vi "VLC - Get Program Location (path).vi"(11 "error in (no error)":errorcluster) -> (6 "VLC path":string, 15 "error out":errorcluster)   [LabVIEW 2016]
uses:
  <vilib>/registry/registry.llb/Registry RtKey.ctl
  <vilib>/registry/registry.llb/Registry SAM.ctl
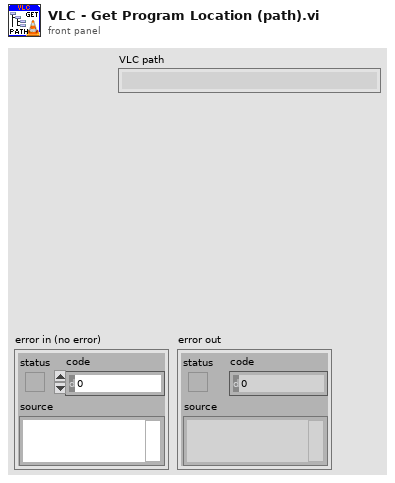
[diagram p1: front panel]
types:
  T1 = typedef "Registry SAM.ctl" = enum32{"KEY_QUERY_VALUE", "KEY_SET_VALUE", "KEY_CREATE_SUB_KEY", "KEY_ENUMERATE_SUB_KEYS", "KEY_NOTIFY", "KEY_CREATE_LINK", "KEY_READ", "KEY_WRITE", "KEY_ALL_ACCESS", "KEY_READ | KEY_WRITE"}
  T2 = typedef "Registry RtKey.ctl" = enum32{"HKEY_CLASSES_ROOT", "HKEY_CURRENT_USER", "HKEY_LOCAL_MACHINE", "HKEY_USERS", "HKEY_PERFORMANCE_DATA", "HKEY_CURRENT_CONFIG", "HKEY_DYN_DATA"}
  T3 = typedef "Registry refnum.ctl" = refnum<k1>
  T4 = cluster{"numValues":i32, "maxValueNameLen":i32, "maxValueDataLen":i32}
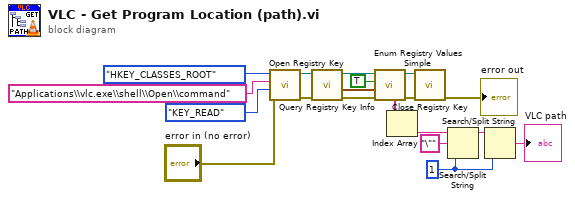
[diagram p0: block diagram]
diagram:
  w5 = 1 ("offset (0)")
  n1 = call <vilib>:"Open Registry Key.vi"("error in (no error)"="error in (no error)", "security access mask (KEY_READ | KEY_WRITE)"=Registry_SAM."KEY_READ", "subkey"="Applications\\vlc.exe\\shell\\Open\\command", "root key (HKEY_LOCAL_MACHINE)"=Registry_RtKey."HKEY_CLASSES_ROOT") -> ("error out"=w15:errorcluster, "refnum out"=w16:T3)  [unwired: 6 in]
  n2 = call <vilib>:"Query Registry Key Info.vi"("error in (no error)"=w15, "refnum"=w16) -> ("error out"=w13:errorcluster, "value info"=w12:T4, "refnum out"=w14:T3)  [unwired: 5 in, 2 out]
  n3 = call <vilib>:"Enum Registry Values Simple.vi"("error in (no error)"=w13, "value info"=w12, "retrieve data? (F)"=TRUE, "refnum"=w14) -> ("error out"=w9:errorcluster, "refnum out"=w10:T3, "String/Binary data"=w8:string[])  [unwired: 2 in, 3 out]
  n4 = Index Array(array=w8) -> (element=w7:string)  [unwired: 1 in]
  n5 = call <vilib>:"Close Registry Key.vi"("error in (no error)"=w9, "refnum"=w10) -> ("error out"=→"error out":errorcluster)  [unwired: 5 in]
  n6 = Search/Split String(string=w7, search string/char (-)="\"", offset (0)=w5) -> (substring before match=w6:string)  [unwired: 2 out]
  n7 = Search/Split String(string=w6, offset (0)=w5) -> (match + rest of string=→"VLC path":string)  [unwired: 1 in, 2 out]
